vi "Store New VI for Category List.vi"(6 "Help Text":string, 8 "error in (no error)":errorcluster, 9 "String":string, 10 "VI Refnum":refnum<vi>, 11 "Configuration in":refnum<class "Configuration.lvclass">) -> (0 "error out":errorcluster, 3 "Configuration out":refnum<class "Configuration.lvclass">)   [LabVIEW 2020, in "Configuration.lvlib" / "Configuration.lvclass"]
uses:
  Configuration.lvclass
  Configuration.lvclass/Configuration.ctl
  Data Retrieved by Lookup Table.ctl
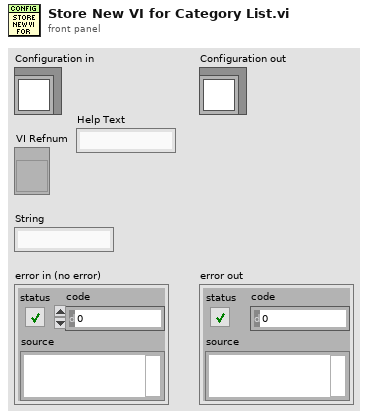
[diagram p1: front panel]
types:
  T1 = typedef "Configuration.lvlib/Configuration.lvclass/Data Retrieved by Lookup Table.ctl" = cluster{"VI Refnum":refnum<vi>, "Help Text":string}
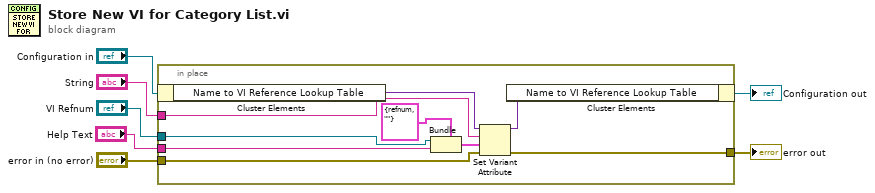
[diagram p0: block diagram]
diagram:
  n1 = in-place {
    in-place-border: "VI Refnum" -> [w11]
    in-place-border: "String" -> [w14]
    in-place-border: "error in (no error)" -> [w13]
    in-place-border: [w12] -> w6
    in-place-border: "Help Text" -> [w10]
    n2 = in-place-cluster #1("Configuration in") -> ("Name to VI Reference Lookup Table"=w16:variant)
    n3 = Bundle(cluster=T1 {"VI Refnum"=refnum, "Help Text"=""} ("output cluster"), "VI Refnum"=w11, "Help Text"=w10) -> (w9:T1)
    n4 = Set Variant Attribute(Variant=w16, name=w14, value=w9, error in=w13) -> (Variant out=w15:variant, error out=w12:errorcluster)  [unwired: 1 out]
    n5 = in-place-cluster #1("Name to VI Reference Lookup Table"=w15) -> (→"Configuration out":refnum<class "Configuration.lvclass">)
  }
  "error out" <- w6
